vi "NewNYPizzaStore.vi"(8 "error in (no error)":errorcluster) -> (0 "error out":errorcluster, 3 "NYPizzaStore":refnum<class "NYPizzaStore.lvclass">)   [LabVIEW 2020, in "FactoryMethod.lvlib" / "PizzaFactoryMethod.lvlib" / "NYPizzaStore.lvclass"]
uses:
  NYPizzaStore.lvclass
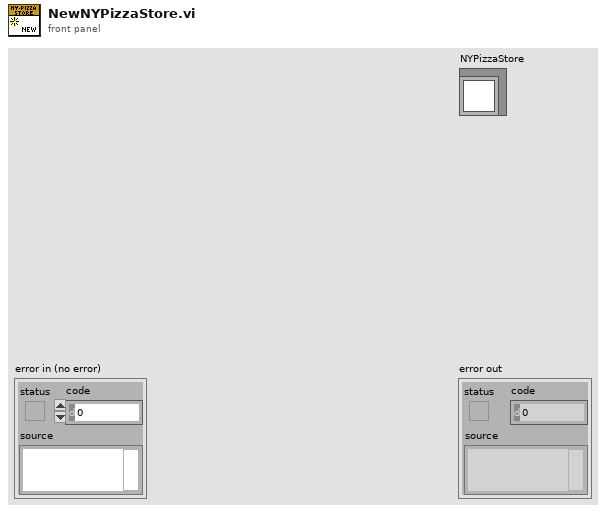
[diagram p1: front panel]
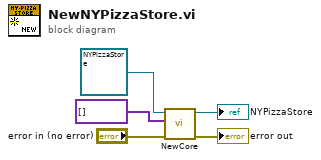
[diagram p0: block diagram]
diagram:
  n1 = call-dynamic "NewCore.vi"("error in (no error)"="error in (no error)", "ParamsArray"=variant[] [], "NYPizzaStore"=refnum<class "NYPizzaStore.lvclass"> refnum) -> ("error out"=→"error out":errorcluster, "NYPizzaStore"=→"NYPizzaStore":refnum<class "NYPizzaStore.lvclass">)  [unwired: 7 in]
